vi "Line Intersection With AABB.vi"(10 "AABB":T1, 11 "Line":T2) -> (3 "Intersects?":bool)   [LabVIEW 2021, in "Collision.lvlib"]
uses:
  Collision.lvlib
  Vector 2D/Vector 2D.lvclass
  Vector 2D/Vector 2D.lvclass/Vector 2D.ctl
  Utility/Typedef/Line.ctl
  Utility/Utility.lvlib
  Utility/Typedef/Axis Aligned Bounding Box.ctl
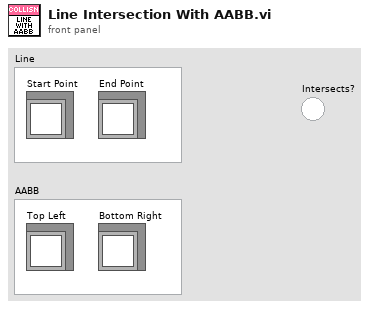
[diagram p1: front panel]
types:
  T1 = typedef "Utility.lvlib/Axis Aligned Bounding Box.ctl" = cluster{"Top Left":refnum<class "Vector 2D.lvclass">, "Bottom Right":refnum<class "Vector 2D.lvclass">}
  T2 = typedef "Utility.lvlib/Line.ctl" = cluster{"Start Point":refnum<class "Vector 2D.lvclass">, "End Point":refnum<class "Vector 2D.lvclass">}
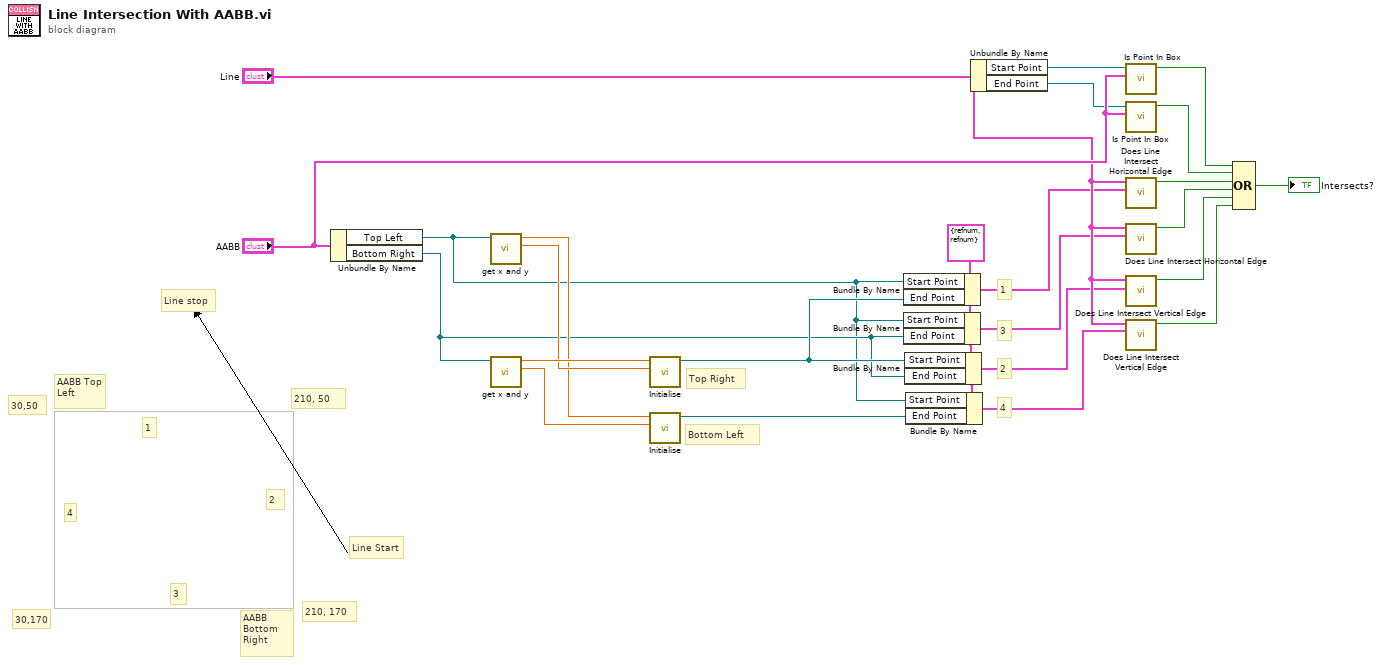
[diagram p0: block diagram]
diagram:
  w19 = T2 {"Start Point"=refnum, "End Point"=refnum} ("Horizontal Edge")
  # "210, 50"
  # "30,170"
  # "210, 170"
  # "30,50"
  # "4"
  # "2"
  # "3"
  # "1"
  # "Bottom Left"
  # "Top Right"
  # "4"
  # "3"
  # "2"
  # "1"
  # "AABB Bottom Right"
  # "AABB Top Left"
  # "Line Start"
  # "Line stop"
  n1 = Unbundle By Name("AABB") -> ("Top Left"=w9:refnum<class "Vector 2D.lvclass">, "Bottom Right"=w10:refnum<class "Vector 2D.lvclass">)
  n2 = call "get x and y.vi"("Vector 2D in"=w9) -> ("y"=w14:sgl, "x"=w13:sgl)  [unwired: 9 in]
  n3 = call "get x and y.vi"("Vector 2D in"=w10) -> ("y"=w12:sgl, "x"=w15:sgl)  [unwired: 9 in]
  n4 = call "Initialise.vi"("y"=w14, "x"=w15) -> ("Vector 2D out"=w11:refnum<class "Vector 2D.lvclass">)  [unwired: 9 in]
  n5 = call "Initialise.vi"("y"=w12, "x"=w13) -> ("Vector 2D out"=w8:refnum<class "Vector 2D.lvclass">)  [unwired: 9 in]
  n6 = Bundle By Name(cluster=w19, "Start Point"=w9, "End Point"=w11) -> (w20:T2)
  n7 = Bundle By Name(cluster=w19, "Start Point"=w9, "End Point"=w10) -> (w18:T2)
  n8 = Bundle By Name(cluster=w19, "Start Point"=w11, "End Point"=w10) -> (w17:T2)
  n9 = Bundle By Name(cluster=w19, "Start Point"=w9, "End Point"=w8) -> (w16:T2)
  n10 = Unbundle By Name("Line") -> ("Start Point"=w22:refnum<class "Vector 2D.lvclass">, "End Point"=w21:refnum<class "Vector 2D.lvclass">)
  n11 = call "Is Point In Box.vi"("AABB"="AABB", "Point"=w22) -> ("In Box?"=w3:bool)  [unwired: 9 in]
  n12 = call "Is Point In Box.vi"("AABB"="AABB", "Point"=w21) -> ("In Box?"=w2:bool)  [unwired: 9 in]
  n13 = call "Does Line Intersect Horizontal Edge.vi"("Horizontal Edge"=w20, "Line"="Line") -> ("Intersects?"=w7:bool)  [unwired: 9 in]
  n14 = call "Does Line Intersect Horizontal Edge.vi"("Horizontal Edge"=w18, "Line"="Line") -> ("Intersects?"=w6:bool)  [unwired: 9 in]
  n15 = call "Does Line Intersect Vertical Edge.vi"("Vertical Edge"=w17, "Line"="Line") -> ("Intersects?"=w5:bool)  [unwired: 9 in]
  n16 = call "Does Line Intersect Vertical Edge.vi"("Vertical Edge"=w16, "Line"="Line") -> ("Intersects?"=w4:bool)  [unwired: 9 in]
  n17 = Compound Arithmetic op=OR(w3, w2, w7, w6, w5, w4) -> (→"Intersects?":bool)
